vi "162-Test QoS 2 Subscription.vi"() -> ()   [LabVIEW 2013]
uses:
  <vilib>/LabVIEW Open Source Project/MQTT Control Packets/Control Packets/CONNACK/Connect Return Code -- enum.ctl
  <vilib>/LabVIEW Open Source Project/MQTT Control Packets/Control Packets/ControlPacket/QualityOfService -- enum.ctl
  source/Server class/Server.lvclass/Server.ctl
  <vilib>/LabVIEW Open Source Project/MQTT Client/Client class/Client.lvclass/Client.ctl
  <vilib>/LabVIEW Open Source Project/MQTT Control Packets/Control Packets/PUBLISH/PUBLISH.lvclass
  source/Server class/Server.lvclass
  <vilib>/LabVIEW Open Source Project/MQTT Connection/MQTT_Base/Base Class/MQTT_Base.lvclass
  <vilib>/LabVIEW Open Source Project/MQTT Client/Client class/Client.lvclass
  <vilib>/LabVIEW Open Source Project/MQTT TCP Connection/MQTT_TCP/Connection/TCPConnection.lvclass
  <vilib>/LabVIEW Open Source Project/MQTT LocalQueue Connection/MQTT_LocalQueue/Connection/LocalQueueConnection.lvclass
  <vilib>/LabVIEW Open Source Project/MQTT Websockets Connection/MQTT_Websockets/Connection/WebsocketsConnection.lvclass
  <vilib>/LabVIEW Open Source Project/MQTT Control Packets/Control Packets/ControlPacket/ControlPacket.lvclass
  <vilib>/LabVIEW Open Source Project/MQTT Control Packets/Control Packets/CONNACK/CONNACK.lvclass
panel:
  out "FAILED":bool
  out "error server":errorcluster
  out "error client sink 2":errorcluster
  out "Random":dbl
  out "received 2":i32
  out "Client Status 2":T1=enum."Server Unavailable"
  out "error client source":errorcluster
  out "NbConnections":u32
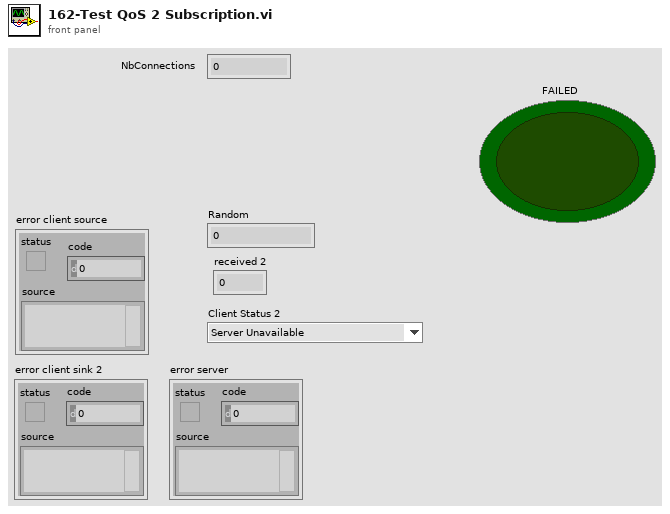
[diagram p1: front panel]
types:
  T1 = typedef "MQTT_Control_Packets.lvlib/CONNACK.lvclass/Connect Return Code -- enum.ctl" = enum16{"Connection accepted", "Unacceptable protocol version", "Identifier Rejected", "Server Unavailable", "Bad Username or Password", "Not Authorized"}
  T2 = typedef "MQTT_Control_Packets.lvlib/ControlPacket.lvclass/QualityOfService -- enum.ctl" = enum16{"0 (At Most Once)", "1 (At Least Once)", "2 (Exactly Once)"}
  T3 = typedef "MQTT Client.lvlib/Client.lvclass/Public Events -- cluster.ctl" = cluster{"Connection Status":refnum<user-event>, "Connected":refnum<user-event>, "Application Message":refnum<user-event>}
  T4 = typedef "MQTT Server.lvlib/Server.lvclass/Public Events -- cluster.ctl" = cluster{"NbConnections":refnum<user-event>}
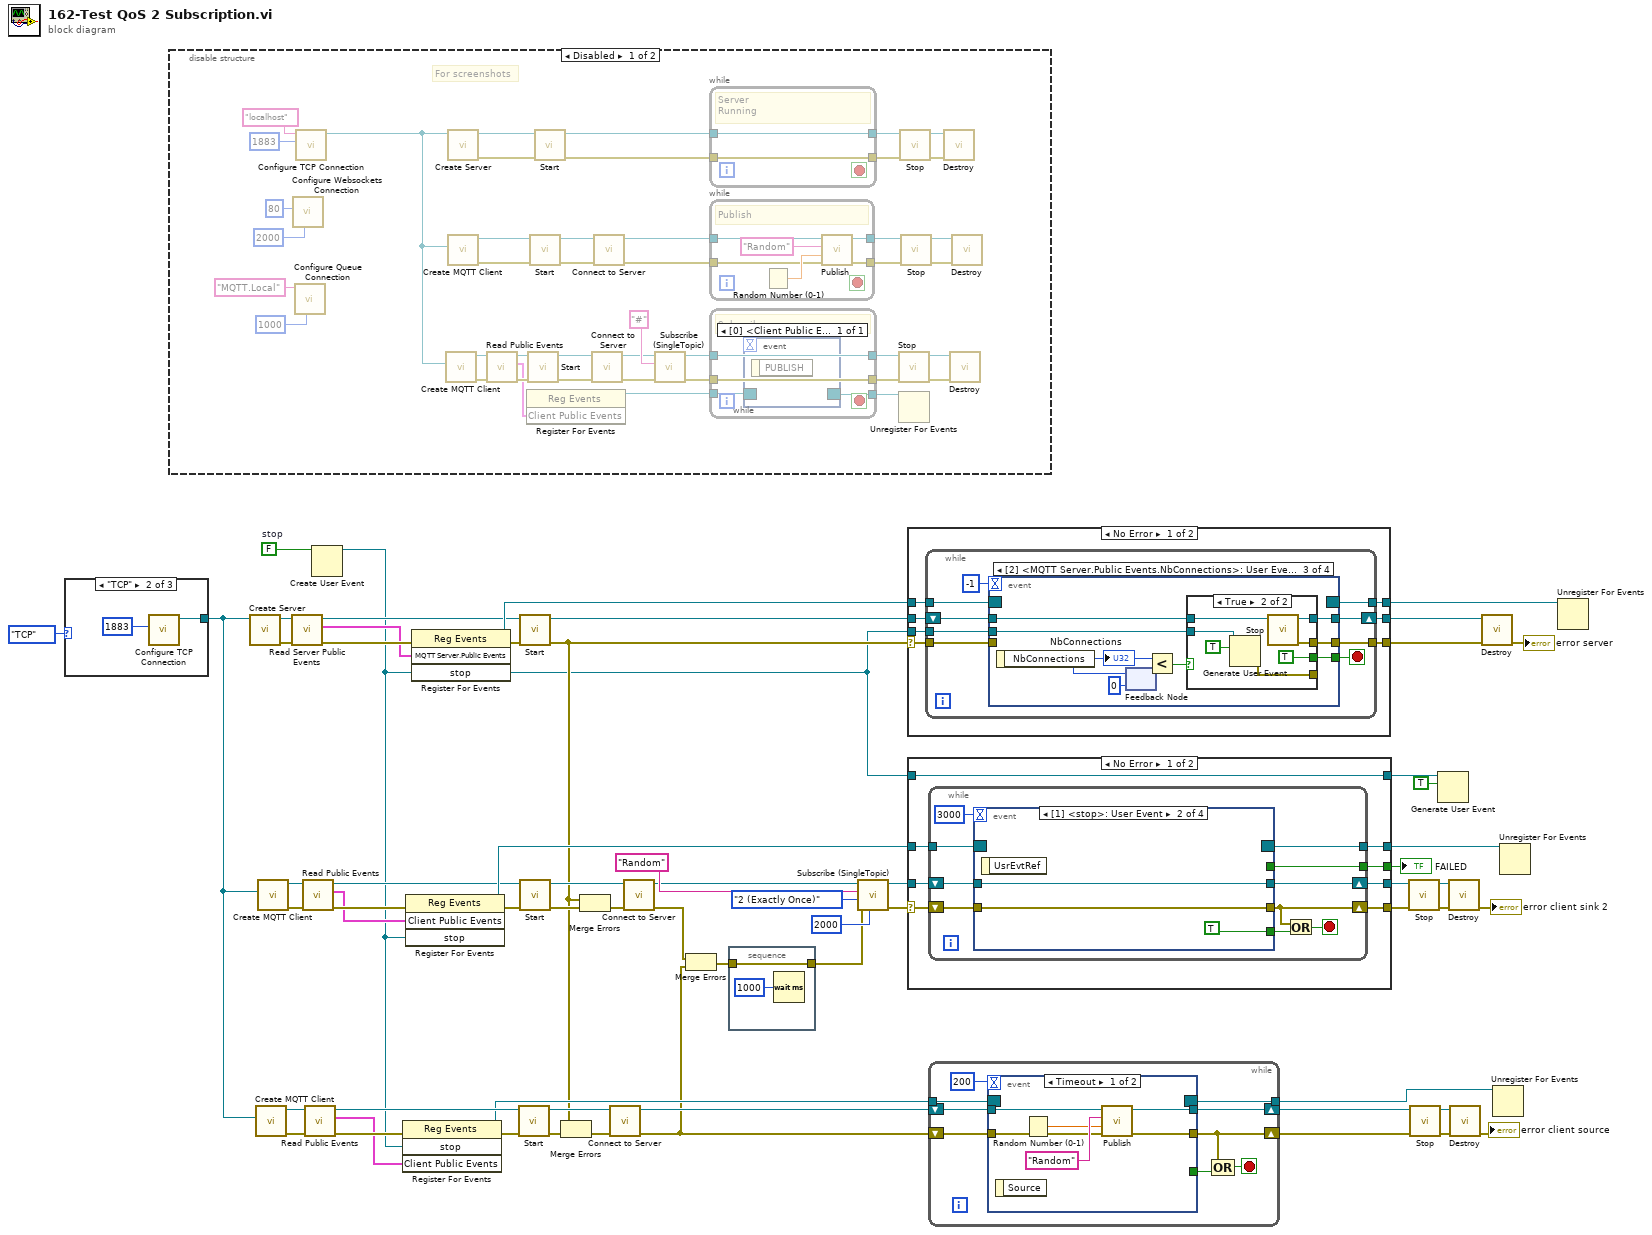
[diagram p0: block diagram]
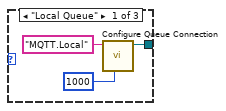
[diagram p2: hidden frame]
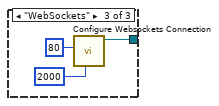
[diagram p3: hidden frame]
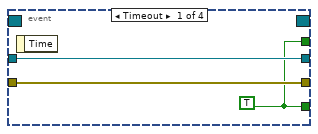
[diagram p5: hidden frame]
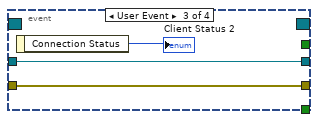
[diagram p6: hidden frame]
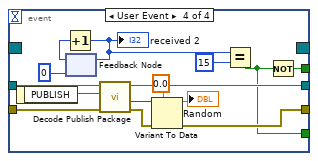
[diagram p7: hidden frame]
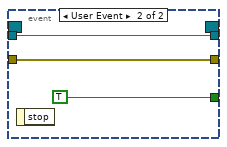
[diagram p9: hidden frame]
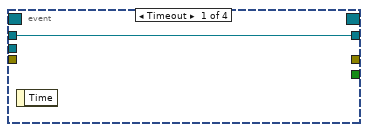
[diagram p10: hidden frame]
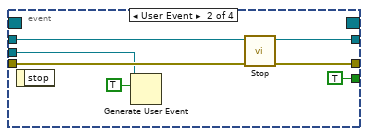
[diagram p11: hidden frame]
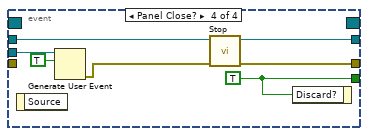
[diagram p13: hidden frame]
diagram:
  w41 = FALSE  # stop
  n1 = case shown="\"TCP\"" enum16{"TCP", "Local Queue", "WebSockets"}."TCP" ("Connection Type") {
    tunnel: [w64 w67 w71] -> w10
    frame "Local Queue" {
      n2 = call <vilib>:"Configure Queue Connection.vi"("timeout (500 ms)"=1000 ("timeout (100ms)"), "Queue Name"="MQTT.Local") -> ("LocalQueueConnection"=w64:refnum<class "LocalQueueConnection.lvclass">)  [unwired: 8 in, 1 out]
    }
    frame "TCP" {
      n3 = call <vilib>:"Configure TCP Connection.vi"("remote port (80)"=u16 1883) -> ("TCPConnection"=w67:refnum<class "TCPConnection.lvclass">)  [unwired: 9 in, 1 out]
    }
    frame "WebSockets" {
      n4 = call <vilib>:"Configure Websockets Connection.vi"("timeout (5000 ms)"=2000 ("timeout (100ms)"), "remote port (80)"=u16 80) -> ("WSConnection"=w71:refnum<class "WebsocketsConnection.lvclass">)  [unwired: 8 in, 1 out]
    }
  }
  n5 = disable-structure shown="Disabled" {
    frame Disabled {
      # "For screenshots"
      n6 = call <vilib>:"Configure Websockets Connection.vi"("timeout (5000 ms)"=2000 ("timeout (100ms)"), "remote port (80)"=u16 80) -> ()  [unwired: 8 in, 2 out]
      n7 = call <vilib>:"Configure Queue Connection.vi"("timeout (500 ms)"=1000 ("timeout (100ms)"), "Queue Name"="MQTT.Local") -> ()  [unwired: 8 in, 2 out]
      n8 = call <vilib>:"Configure TCP Connection.vi"("remote port (80)"=u16 1883, "address (localhost)"="localhost" ("Topic Filter")) -> ("TCPConnection"=w77:refnum<class "TCPConnection.lvclass">)  [unwired: 8 in, 1 out]
      n9 = call <vilib>:"Create MQTT Client.vi"("Connection Configuration"=w77) -> ("error out"=w83:errorcluster, "Client out"=w85:refnum<class "Client.lvclass">)  [unwired: 9 in]
      n10 = call "Create Server.vi"("Connection Configuration"=w77) -> ("error out"=w108:errorcluster, "Server"=w107:refnum<class "Server.lvclass">)  [unwired: 9 in]
      n11 = call <vilib>:"Create MQTT Client.vi"("Connection Configuration"=w77) -> ("error out"=w105:errorcluster, "Client out"=w106:refnum<class "Client.lvclass">)  [unwired: 9 in]
      n12 = call <vilib>:"Read Public Events.vi"("error in (no error)"=w83, "Client in"=w85) -> ("error out"=w82:errorcluster, "Client Public Events"=w81:T3, "Client out"=w84:refnum<class "Client.lvclass">)  [unwired: 7 in]
      n13 = register-events(w81) -> (reference out=w80:refnum<event-registration>)  [unwired: 2 in, 1 out]
      n14 = call <vilib>:"Start.vi"("error in (no error)"=w82, "MQTT_Base in"=w84) -> ("error out"=w100:errorcluster, "MQTT_Base out"=w101:refnum<class "Client.lvclass">)  [unwired: 7 in, 1 out]
      n15 = call <vilib>:"Start.vi"("error in (no error)"=w105, "MQTT_Base in"=w106) -> ("error out"=w112:errorcluster, "MQTT_Base out"=w111:refnum<class "Client.lvclass">)  [unwired: 7 in, 1 out]
      n16 = call <vilib>:"Start.vi"("error in (no error)"=w108, "MQTT_Base in"=w107) -> ("error out"=w92:errorcluster, "MQTT_Base out"=w94:refnum<class "Server.lvclass">)  [unwired: 7 in, 1 out]
      n17 = call <vilib>:"Connect to Server.vi"("error in (no error)"=w100, "Client in"=w101) -> ("error out"=w88:errorcluster, "Client out"=w89:refnum<class "Client.lvclass">)  [unwired: 6 in, 2 out]
      n18 = call <vilib>:"Connect to Server.vi"("error in (no error)"=w112, "Client in"=w111) -> ("error out"=w96:errorcluster, "Client out"=w99:refnum<class "Client.lvclass">)  [unwired: 6 in, 2 out]
      n19 = call <vilib>:"Subscribe (SingleTopic).vi"("error in (no error)"=w88, "Topic Filter"="#", "MQTT_Base in"=w89) -> ("error out"=w86:errorcluster, "MQTT_Base out"=w87:refnum<class "Client.lvclass">)  [unwired: 6 in, 1 out]
      n20 = while {
        tunnel: [w126] -> w95
        tunnel: w94 -> [w126]
        tunnel: w92 -> [w125]
        tunnel: [w125] -> w93
        stop <- _ stop-if-true
        # "Server\nRunning"
      }
      n21 = while {
        tunnel: w99 -> [w122]
        tunnel: [w121] -> w98
        tunnel: [w120] -> w97
        tunnel: w96 -> [w119]
        stop <- _ stop-if-true
        # "Publish"
        n22 = Random Number (0-1)() -> (number: 0 to 1=w124:dbl)
        n23 = call <vilib>:"Publish.vi"("error in (no error)"=w119, "Payload"=w124, "Topic Name (empty: Payload name)"="Random", "Client in"=w122) -> ("error out"=w120:errorcluster, "Client out"=w121:refnum<class "Client.lvclass">)  [unwired: 5 in, 1 out]
      }
      n24 = while {
        tunnel: [w118] -> w90
        tunnel: w87 -> [w118]
        tunnel: w86 -> [w117]
        tunnel: [w117] -> w91
        tunnel: w80 -> [w116]
        tunnel: [w115] -> w79
        stop <- _ stop-if-true
        # "Subscribe"
        n25 = event shown="[0] <Client Public Events.Application Message>: User Event" {
          selector: w116 -> [_]
          dyn-events: [_] -> w115
          timeout: _ -> [_]
          event User Event {
            n26 = event-data() -> ()  [unwired: 1 in, 1 out]
          }
        }
      }
      n27 = call <vilib>:"Stop.vi"("error in (no error)"=w91, "MQTT_Base in"=w90) -> ("error out"=w103:errorcluster, "MQTT_Base out"=w104:refnum<class "Client.lvclass">)  [unwired: 7 in, 1 out]
      n28 = Unregister For Events(event registration refnum=w79) -> ()  [unwired: 1 in, 1 out]
      n29 = call <vilib>:"Stop.vi"("error in (no error)"=w93, "MQTT_Base in"=w95) -> ("error out"=w114:errorcluster, "MQTT_Base out"=w113:refnum<class "Server.lvclass">)  [unwired: 7 in, 1 out]
      n30 = call <vilib>:"Stop.vi"("error in (no error)"=w97, "MQTT_Base in"=w98) -> ("error out"=w110:errorcluster, "MQTT_Base out"=w109:refnum<class "Client.lvclass">)  [unwired: 7 in, 1 out]
      n31 = call <vilib>:"Destroy.vi"("error in (no error)"=w114, "MQTT_Base in"=w113) -> ()  [unwired: 8 in, 2 out]
      n32 = call <vilib>:"Destroy.vi"("error in (no error)"=w103, "MQTT_Base in"=w104) -> ()  [unwired: 8 in, 2 out]
      n33 = call <vilib>:"Destroy.vi"("error in (no error)"=w110, "MQTT_Base in"=w109) -> ()  [unwired: 8 in, 2 out]
    }
    frame Enabled {
    }
  }
  n34 = call "Create Server.vi"("Connection Configuration"=w10) -> ("error out"=w61:errorcluster, "Server"=w62:refnum<class "Server.lvclass">)  [unwired: 9 in]
  n35 = call <vilib>:"Create MQTT Client.vi"("Connection Configuration"=w10) -> ("error out"=w50:errorcluster, "Client out"=w49:refnum<class "Client.lvclass">)  [unwired: 9 in]
  n36 = call <vilib>:"Create MQTT Client.vi"("Connection Configuration"=w10) -> ("error out"=w20:errorcluster, "Client out"=w19:refnum<class "Client.lvclass">)  [unwired: 9 in]
  n37 = call "Read Server Public Events.vi"("error in (no error)"=w61, "Server in"=w62) -> ("error out"=w60:errorcluster, "MQTT Server.Public Events"=w59:T4, "Server out"=w56:refnum<class "Server.lvclass">)  [unwired: 7 in]
  n38 = call <vilib>:"Read Public Events.vi"("error in (no error)"=w20, "Client in"=w19) -> ("error out"=w29:errorcluster, "Client Public Events"=w28:T3, "Client out"=w21:refnum<class "Client.lvclass">)  [unwired: 7 in]
  n39 = call <vilib>:"Read Public Events.vi"("error in (no error)"=w50, "Client in"=w49) -> ("error out"=w40:errorcluster, "Client Public Events"=w36:T3, "Client out"=w48:refnum<class "Client.lvclass">)  [unwired: 7 in]
  n40 = Create User Event(user event datatype=w41) -> (user event=w2:refnum<user-event>)  [unwired: 1 in, 1 out]
  n41 = register-events(error in=w40, w2, w36) -> (reference out=w38:refnum<event-registration>, error out=w39:errorcluster)  [unwired: 1 in]
  n42 = register-events(error in=w29, w28, w2) -> (reference out=w31:refnum<event-registration>, error out=w30:errorcluster)  [unwired: 1 in]
  n43 = register-events(error in=w60, w59, w2) -> (reference out=w58:refnum<event-registration>, error out=w54:errorcluster)  [unwired: 1 in]
  n44 = call <vilib>:"Start.vi"("error in (no error)"=w39, "MQTT_Base in"=w48) -> ("error out"=w46:errorcluster, "MQTT_Base out"=w47:refnum<class "Client.lvclass">)  [unwired: 7 in, 1 out]
  n45 = call <vilib>:"Start.vi"("error in (no error)"=w54, "MQTT_Base in"=w56) -> ("error out"=w16:errorcluster, "MQTT_Base out"=w55:refnum<class "Server.lvclass">)  [unwired: 7 in, 1 out]
  n46 = call <vilib>:"Start.vi"("error in (no error)"=w30, "MQTT_Base in"=w21) -> ("error out"=w23:errorcluster, "MQTT_Base out"=w22:refnum<class "Client.lvclass">)  [unwired: 7 in, 1 out]
  n47 = Merge Errors(w16, w46) -> (w51:errorcluster)
  n48 = Merge Errors(w16, w23) -> (w18:errorcluster)
  n49 = call <vilib>:"Connect to Server.vi"("error in (no error)"=w51, "Client in"=w47) -> ("error out"=w4:errorcluster, "Client out"=w5:refnum<class "Client.lvclass">)  [unwired: 6 in, 2 out]
  n50 = call <vilib>:"Connect to Server.vi"("error in (no error)"=w18, "Client in"=w22) -> ("error out"=w7:errorcluster, "Client out"=w26:refnum<class "Client.lvclass">)  [unwired: 6 in, 2 out]
  n51 = Merge Errors(w7, w4) -> (w42:errorcluster)
  n52 = stacked-sequence {
    tunnel: [w127] -> w6
    tunnel: w42 -> [w127]
    frame #0 {
      n53 = Wait (ms)(milliseconds to wait=u32 1000) -> ()  [unwired: 1 out]
    }
  }
  n54 = call <vilib>:"Subscribe (SingleTopic).vi"("timeout (100ms)"=2000, "error in (no error)"=w6, "QoS"=QualityOfService_--_enum."2 (Exactly Once)" ("QoS Subscription"), "Topic Filter"="Random", "MQTT_Base in"=w26) -> ("error out"=w15:errorcluster, "MQTT_Base out"=w33:refnum<class "Client.lvclass">)  [unwired: 4 in, 1 out]
  n55 = case shown="No Error" w16 {
    selector: w16 -> [w129 w177]
    tunnel: w55 -> [w135 w179]
    tunnel: [w134 w179] -> w63
    tunnel: w58 -> [w133 w178]
    tunnel: [w132 w178] -> w57
    tunnel: [w131 w177] -> w53
    tunnel: w2 -> [w130 _]
    frame No Error {
      n56 = while {
        shift-right: [w141] -> w134
        shift-left: w135 -> [w143]
        tunnel: w133 -> [w140]
        tunnel: [w139] -> w132
        tunnel: [w138] -> w131
        tunnel: w130 -> [w137]
        tunnel: w129 -> [w136]
        stop <- w142 stop-if-true
        n57 = event shown="[2] <MQTT Server.Public Events.NbConnections>: User Event" {
          selector: w140 -> [_ _ _ _]
          dyn-events: [_ _ _ _] -> w139
          timeout: -1 -> [_ _ _ _]
          tunnel: w143 -> [w145 w152 w158 w176]
          tunnel: [_ TRUE ("Discard?") w154 w175] -> w142
          tunnel: [w145 w151 w157 w174] -> w141
          tunnel: [_ w150 w156 w173] -> w138
          tunnel: w137 -> [_ w146 w153 w172]
          tunnel: w136 -> [_ w148 _ _]
          event Timeout {
            n58 = event-data() -> ()  [unwired: 1 in, 1 out]
          }
          event User Event {
            n59 = event-data() -> ()  [unwired: 1 in, 1 out]
            n60 = Generate User Event(user event=w146, event data cluster=TRUE ("event data")) -> ()  [unwired: 2 in, 2 out]
            n61 = call <vilib>:"Stop.vi"("error in (no error)"=w148, "MQTT_Base in"=w152) -> ("error out"=w150:errorcluster, "MQTT_Base out"=w151:refnum<class "Server.lvclass">)  [unwired: 7 in, 1 out]
          }
          event User Event {
            n62 = event-data() -> ("NbConnections"=w160:u32)  [unwired: 1 in]
            "NbConnections" <- w160
            n63 = feedback #1(u32 0 ("NbConnections")) -> (w159:u32)
            n64 = feedback-in #1(w160) -> ()
            n65 = Less?(x=w160, y=w159) -> (x < y?=w155:bool)
            n66 = case shown="True" w155 {
              tunnel: w158 -> [w162 w169]
              tunnel: [w162 w168] -> w157
              tunnel: [_ w167] -> w156
              tunnel: [_ TRUE] -> w154
              tunnel: w153 -> [_ w164]
              tunnel: [_ w163] -> _
              frame False {
              }
              frame True {
                n67 = Generate User Event(user event=w164, event data cluster=TRUE ("event data")) -> (error out=w163:errorcluster)  [unwired: 2 in, 1 out]
                n68 = call <vilib>:"Stop.vi"("MQTT_Base in"=w169) -> ("error out"=w167:errorcluster, "MQTT_Base out"=w168:refnum<class "Server.lvclass">)  [unwired: 8 in, 1 out]
              }
            }
          }
          event Panel Close? {
            w175 = TRUE ("Discard?")
            n69 = event-data() -> ()  [unwired: 1 in, 1 out]
            n70 = Generate User Event(user event=w172, event data cluster=TRUE ("event data")) -> (error out=w170:errorcluster)  [unwired: 2 in, 1 out]
            n71 = call <vilib>:"Stop.vi"("error in (no error)"=w170, "MQTT_Base in"=w176) -> ("error out"=w173:errorcluster, "MQTT_Base out"=w174:refnum<class "Server.lvclass">)  [unwired: 7 in, 1 out]
            n72 = event-data("Discard?"=w175) -> ()  [unwired: 1 in, 1 out]
          }
        }
      }
    }
    frame Error {
    }
  }
  n73 = case shown="No Error" w15 {
    selector: w15 -> [w182 w223]
    tunnel: w31 -> [w187 w225]
    tunnel: [w186 w225] -> w32
    tunnel: w33 -> [w185 w224]
    tunnel: [w184 w224] -> w34
    tunnel: [w183 w223] -> w35
    tunnel: [w181 _] -> w9
    tunnel: w2 -> [w180 w222]
    tunnel: [w180 w222] -> w1
    frame No Error {
      n74 = while {
        tunnel: w187 -> [w197]
        tunnel: [w196] -> w186
        shift-right: [w194] -> w184
        shift-left: w185 -> [w195]
        shift-right: [w191] -> w183
        shift-left: w182 -> [w193]
        tunnel: [w188] -> w181
        stop <- w192 stop-if-true
        n75 = event shown="[1] <stop>: User Event" {
          selector: w197 -> [_ _ _ _]
          dyn-events: [_ _ _ _] -> w196
          timeout: 3000 -> [_ _ _ _]
          tunnel: w195 -> [w200 w202 w205 w221]
          tunnel: [w200 w202 w205 w217] -> w194
          tunnel: [w199 w201 w204 w212] -> w191
          tunnel: w193 -> [w199 w201 w204 w216]
          tunnel: [w198 TRUE _ w208] -> w190
          tunnel: [w198 _ _ w207] -> w188
          event Timeout {
            w198 = TRUE
            n76 = event-data() -> ()  [unwired: 1 in, 1 out]
          }
          event User Event {
            n77 = event-data() -> ()  [unwired: 1 in, 1 out]
          }
          event User Event {
            n78 = event-data() -> ("Connection Status"=→"Client Status 2":T1)  [unwired: 1 in]
          }
          event User Event {
            n79 = event-data() -> ("PUBLISH"=w211:refnum<class "PUBLISH.lvclass">)  [unwired: 1 in]
            n80 = feedback #2(0 ("received")) -> (w214:i32)
            n81 = Increment(x=w214) -> (x+1=w210:i32)
            "received 2" <- w210
            n82 = feedback-in #2(w210) -> ()
            n83 = call <vilib>:"Decode Publish Package.vi"("error in (no error)"=w216, "PUBLISH"=w211, "MQTT_Base in"=w221) -> ("error out"=w213:errorcluster, "Payload"=w220:variant, "MQTT_Base out"=w217:refnum<class "Client.lvclass">)  [unwired: 5 in, 1 out]
            n84 = Variant To Data(error in=w213, type=0.0, Variant=w220) -> (data=→"Random":dbl, error out=w212:errorcluster)
            n85 = Equal?(x=w210, y=15) -> (x = y?=w208:bool)
            n86 = Not(x=w208) -> (.not. x?=w207:bool)
          }
        }
        n87 = Or(x=w191, y=w190) -> (x .or. y?=w192:bool)
      }
    }
    frame Error {
    }
  }
  "FAILED" <- w9
  n88 = while {
    shift-right: [w233] -> w45
    shift-left: w5 -> [w234]
    shift-right: [w226] -> w37
    shift-left: w4 -> [w232]
    tunnel: w38 -> [w230]
    tunnel: [w228] -> w14
    stop <- w231 stop-if-true
    n89 = event shown="[0] Timeout" {
      selector: w230 -> [_ _]
      dyn-events: [_ _] -> w228
      timeout: 200 -> [_ _]
      tunnel: w234 -> [w238 w241]
      tunnel: [w235 w241] -> w233
      tunnel: w232 -> [w237 w242]
      tunnel: [w236 w242] -> w226
      tunnel: [_ TRUE] -> w229
      event Timeout {
        n90 = event-data() -> ()  [unwired: 1 in, 1 out]
        n91 = Random Number (0-1)() -> (number: 0 to 1=w239:dbl)
        n92 = call <vilib>:"Publish.vi"("error in (no error)"=w237, "Payload"=w239, "Topic Name (empty: Payload name)"="Random", "Client in"=w238) -> ("error out"=w236:errorcluster, "Client out"=w235:refnum<class "Client.lvclass">)  [unwired: 5 in, 1 out]
      }
      event User Event {
        n93 = event-data() -> ()  [unwired: 1 in, 1 out]
      }
    }
    n94 = Compound Arithmetic op=OR(w226, w229) -> (w231:bool)
  }
  n95 = call <vilib>:"Stop.vi"("error in (no error)"=w35, "MQTT_Base in"=w34) -> ("error out"=w24:errorcluster, "MQTT_Base out"=w25:refnum<class "Client.lvclass">)  [unwired: 7 in, 1 out]
  n96 = call <vilib>:"Stop.vi"("error in (no error)"=w37, "MQTT_Base in"=w45) -> ("error out"=w43:errorcluster, "MQTT_Base out"=w44:refnum<class "Client.lvclass">)  [unwired: 7 in, 1 out]
  n97 = Generate User Event(user event=w1, event data cluster=TRUE ("event data")) -> ()  [unwired: 2 in, 2 out]
  n98 = call <vilib>:"Destroy.vi"("error in (no error)"=w24, "MQTT_Base in"=w25) -> ("error out"=→"error client sink 2":errorcluster)  [unwired: 8 in, 1 out]
  n99 = call <vilib>:"Destroy.vi"("error in (no error)"=w43, "MQTT_Base in"=w44) -> ("error out"=→"error client source":errorcluster)  [unwired: 8 in, 1 out]
  n100 = call <vilib>:"Destroy.vi"("error in (no error)"=w53, "MQTT_Base in"=w63) -> ("error out"=→"error server":errorcluster)  [unwired: 8 in, 1 out]
  n101 = Unregister For Events(event registration refnum=w14) -> ()  [unwired: 1 in, 1 out]
  n102 = Unregister For Events(event registration refnum=w32) -> ()  [unwired: 1 in, 1 out]
  n103 = Unregister For Events(event registration refnum=w57) -> ()  [unwired: 1 in, 1 out]
